vi "center_detector.vi"(2 "Image":T1, 3 "size_m":dbl, 4 "size_px":dbl) -> (0 "y":dbl, 1 "x":dbl)   [LabVIEW 2019]
uses:
  <vilib>/vision/Image Controls.llb/IMAQ Image.ctl
  <vilib>/vision/NI_Vision_Development_Module.lvlib
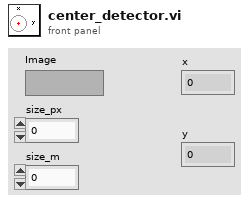
[diagram p1: front panel]
types:
  T1 = typedef "IMAQ Image.ctl" = refnum<image>
  T2 = cluster{"Global Rectangle":i32[], "Contours":cluster{"ID":enum32{"External", "Internal"}, "Type":u32, "Coordinates":i32[]}[]}
  T3 = cluster{"Position":cluster{"X":sgl, "Y":sgl}, "Radius":dbl, "Score":dbl}[]
  T4 = cluster{"Position":cluster{"X":sgl, "Y":sgl}, "Radius":dbl, "Score":dbl}
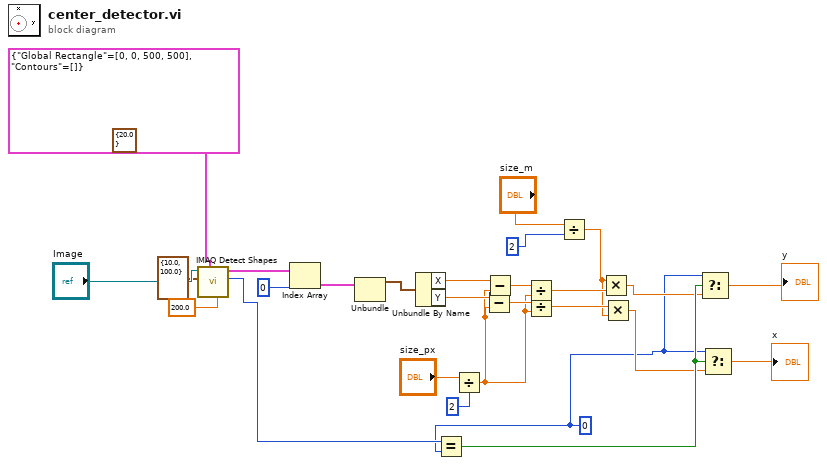
[diagram p0: block diagram]
diagram:
  w3 = 0
  (unwired) cluster{"Min Radius":dbl} {"Min Radius"=20.0} ("Circle Descriptor")
  n1 = call-poly "IMAQ Detect Shapes"("Minimum match score"=200.0, "ROI Descriptor"=T2 {"Global Rectangle"=[0, 0, 500, 500], "Contours"=[]}, "Circle Descriptor"=cluster{"Min Radius":dbl, "Max Radius":dbl} {"Min Radius"=10.0, "Max Radius"=100.0}, "Image"="Image") -> ("Number of Matches Returned"=w7:i32, "Circles"=w23:T3)  [unwired: 5 in, 1 out]
  n2 = Index Array(array=w23, index=0) -> (element=w21:T4)
  n3 = Unbundle(w21) -> ("Position"=w20:cluster{"X":sgl, "Y":sgl})  [unwired: 2 out]
  n4 = Unbundle By Name(w20) -> ("X"=w16:sgl, "Y"=w17:sgl)
  n5 = Equal?(x=w7, y=w3) -> (x = y?=w6:bool)
  n6 = Divide(x="size_px", y=2) -> (x/y=w13:dbl)
  n7 = Subtract(x=w17, y=w13) -> (x-y=w14:dbl)
  n8 = Subtract(x=w16, y=w13) -> (x-y=w15:dbl)
  n9 = Divide(x=w15, y=w13) -> (x/y=w12:dbl)
  n10 = Divide(x=w14, y=w13) -> (x/y=w11:dbl)
  n11 = Divide(x="size_m", y=2) -> (x/y=w10:dbl)
  n12 = Multiply(x=w10, y=w12) -> (x*y=w5:dbl)
  n13 = Multiply(x=w11, y=w10) -> (x*y=w4:dbl)
  n14 = Select(t=w3, s=w6, f=w5) -> (s? t:f=→"y":dbl)
  n15 = Select(t=w3, s=w6, f=w4) -> (s? t:f=→"x":dbl)
